vi "Toggle Main.vi"() -> ()   [LabVIEW 2020, in "VolatusScratch.lvlib"]
uses:
  VolatusScratch.lvlib
  Volatus/MessageQ/MessageQ.lvclass/MessageQ.ctl
  VolatusConfig/VolatusConfig/VolatusConfig.lvclass
  VolatusConfig/System/System.lvclass
  VolatusConfig/Cluster/Cluster.lvclass
  VolatusConfig/Node/Node.lvclass
  Volatus/MessageQ/MessageQ.lvclass
  lv-vecto/Vecto/Node Config/TCP Messaging Info.ctl
  lv-vecto/VectoConfig/VectoConfig.lvlib
  VolatusConfig/Endpoint.ctl
  VolatusConfig/VolatusConfig.lvlib
  VolatusConfig/VolatusConfigElement/VolatusConfigElement.lvclass
  lv-cdm/CDM-Config/Config Element/Config Element.lvclass
  Volatus/Volatus Core/Volatus Core.lvclass
  VolatusConfig/Task/Task.lvclass
  C:/dev/lv20CE/relink/lv-volatus/VolatusConfig/VolatusConfigElement/VolatusConfigElement.lvclass
panel:
  out "error out":errorcluster
  out "Max Size":i32
  out "Depth":i32
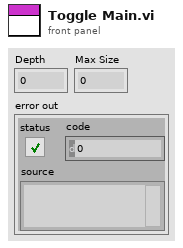
[diagram p1: front panel]
types:
  T1 = typedef "VolatusConfig.lvlib/Endpoint.ctl" = cluster{"Address":string, "Port":u16}
  T2 = typedef "VectoConfig.lvlib/TCP Messaging Info.ctl" = cluster{"Address":string, "Port":u16, "Server (Client)":bool}
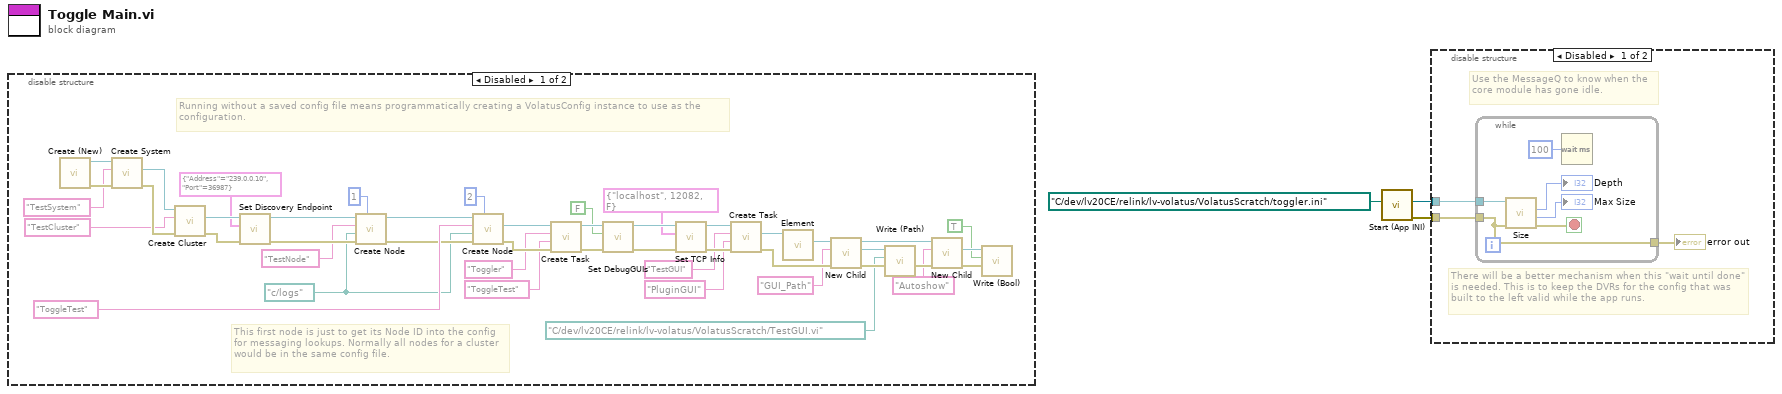
[diagram p0: block diagram]
diagram:
  n1 = disable-structure shown="Disabled" {
    frame Disabled {
      w21 = path "c:/logs"
      # "This first node is just to get its Node ID into the config for messaging lookups. Normally all nodes for a cluster would be in the same config file."
      # "Running without a saved config file means programmatically creating a VolatusConfig instance to use as the configuration."
      n2 = call "Create (New).vi"() -> ("error out"=w44:errorcluster, "VolatusConfig out"=w43:refnum<class "VolatusConfig.lvclass">)  [unwired: 10 in]
      n3 = call "Create System.vi"("error in (no error)"=w44, "System Name"="TestSystem", "VolatusConfig in"=w43) -> ("error out"=w45:errorcluster, "System"=w41:refnum<class "System.lvclass">)  [unwired: 6 in, 1 out]
      n4 = call "Create Cluster.vi"("error in (no error)"=w45, "Cluster Name"="TestCluster" ("System Name"), "System in"=w41) -> ("error out"=w26:errorcluster, "Cluster"=w27:refnum<class "Cluster.lvclass">)  [unwired: 6 in, 1 out]
      n5 = call "Set Discovery Endpoint.vi"("error in (no error)"=w26, "Discovery Endpoint"=T1 {"Address"="239.0.0.10", "Port"=36987}, "Cluster in"=w27) -> ("error out"=w46:errorcluster, "Cluster out"=w23:refnum<class "Cluster.lvclass">)  [unwired: 7 in]
      n6 = call "Create Node.vi"("Node ID"=u32 1, "error in (no error)"=w46, "Event Log Folder"=w21, "Node Name"="TestNode", "Cluster in"=w23) -> ("error out"=w24:errorcluster, "Cluster out"=w22:refnum<class "Cluster.lvclass">)  [unwired: 4 in, 1 out]
      n7 = call "Create Node.vi"("Node ID"=u32 2, "error in (no error)"=w24, "Event Log Folder"=w21, "Node Name"="ToggleTest" ("System Name"), "Cluster in"=w22) -> ("error out"=w38:errorcluster, "Node"=w39:refnum<class "Node.lvclass">)  [unwired: 4 in, 1 out]
      n8 = call "Create Task.vi"("error in (no error)"=w38, "Task Type"="ToggleTest", "Task Name"="Toggler", "Node in"=w39) -> ("error out"=w32:errorcluster, "Node out"=w34:refnum<class "Node.lvclass">)  [unwired: 5 in, 1 out]
      n9 = call "Set DebugGUIs.vi"("error in (no error)"=w32, "DebugGUIs"=FALSE, "Node in"=w34) -> ("error out"=w29:errorcluster, "Node out"=w30:refnum<class "Node.lvclass">)  [unwired: 7 in]
      n10 = call "Set TCP Info.vi"("error in (no error)"=w29, "TCP Messaging Info"=T2 {"Address"="localhost", "Port"=12082, "Server (Client)"=FALSE}, "Node in"=w30) -> ("error out"=w17:errorcluster, "Node out"=w18:refnum<class "Node.lvclass">)  [unwired: 7 in]
      n11 = call "Create Task.vi"("error in (no error)"=w17, "Task Type"="PluginGUI", "Task Name"="TestGUI", "Node in"=w18) -> ("error out"=w47:errorcluster, "Task"=w14:refnum<class "Task.lvclass">)  [unwired: 5 in, 1 out]
      n12 = call "Element.vi"("VolatusConfigElement in"=w14) -> ("Element"=w13:refnum<class "Config Element.lvclass">)  [unwired: 9 in, 1 out]
      n13 = call "New Child.vi"("error in (no error)"=w47, "Child Name"="GUI_Path", "Config Element in"=w13) -> ("error out"=w11:errorcluster, "New Child"=w10:refnum<class "Config Element.lvclass">, "Config Element out"=w7:refnum<class "Config Element.lvclass">)  [unwired: 6 in]
      n14 = call "Write (Path).vi"("error in (no error)"=w11, "Path Value"=path "C:/dev/lv20CE/relink/lv-volatus/VolatusScratch/TestGUI.vi", "Config Element in"=w10) -> ("error out"=w48:errorcluster)  [unwired: 7 in, 1 out]
      n15 = call "New Child.vi"("error in (no error)"=w48, "Child Name"="Autoshow", "Config Element in"=w7) -> ("error out"=w6:errorcluster, "New Child"=w5:refnum<class "Config Element.lvclass">)  [unwired: 6 in, 1 out]
      n16 = call "Write (Bool).vi"("error in (no error)"=w6, "Bool Value"=TRUE, "Config Element in"=w5) -> ()  [unwired: 7 in, 2 out]
    }
    frame Enabled {
    }
  }
  n17 = call "Start (App INI).vi"("INI Path (Default)"=path "C:/dev/lv20CE/relink/lv-volatus/VolatusScratch/toggler.ini") -> ("error out"=w2:errorcluster, "MessageQ"=w3:refnum<class "MessageQ.lvclass">)  [unwired: 9 in]
  n18 = disable-structure shown="Disabled" {
    disable-tunnel: w3 -> [w51 _]
    disable-tunnel: w2 -> [w50 _]
    frame Disabled {
      # "There will be a better mechanism when this \"wait until done\" is needed. This is to keep the DVRs for the config that was built to the left valid while the app runs."
      # "Use the MessageQ to know when the core module has gone idle."
      n19 = while {
        tunnel: w51 -> [w57]
        tunnel: w50 -> [w52]
        tunnel: [w52] -> w49
        stop <- w54 stop-if-true
        n20 = call "Size.vi"("error in (no error)"=w52, "MessageQ in"=w57) -> ("error out"=w54:errorcluster, "Max Size"=→"Max Size":i32, "Depth"=→"Depth":i32)  [unwired: 6 in, 1 out]
        n21 = Wait (ms)(milliseconds to wait=u32 100) -> ()  [unwired: 1 out]
      }
      "error out" <- w49
    }
    frame Enabled {
    }
  }
